vi "OSA_example_XYarray.vi"() -> ()   [LabVIEW 2010]
doc: "Example of how to create the X-data if not present after acquisition."
uses:
  _OSA_class/OSA.lvclass
  _OSA_class/typeDef/acq_dataType.ctl
  _misc/Thorlabs_FTS_misc.llb/graph_spectrum.ctl
  OSA20X_misc.lvlib
panel:
  out "timeOut":bool
  in  "X-UNIT":T1(ring)=enum."NM_VAC"
  out "Intensity Graph spectrum":T2
  in  "virtual OSA":bool=TRUE
  out "X,Y (row 0,1)":sgl[][](array[numeric])
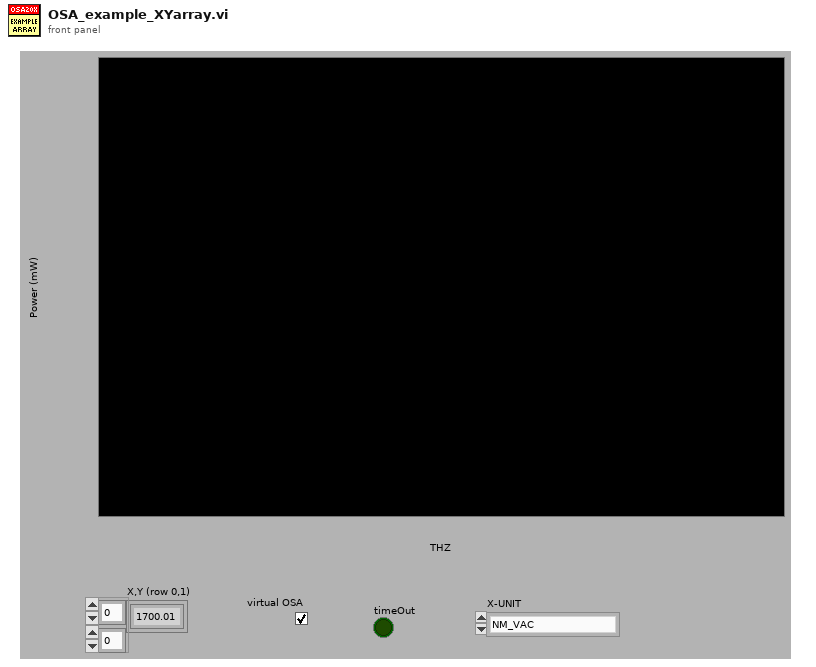
[diagram p1: front panel]
types:
  T1 = enum16{"WAVENR/CM", "EV", "THZ", "NM_AIR", "NM_VAC"}
  T2 = typedef "OSA20X_misc.lvlib/graph_spectrum.ctl" = i32[][]
  T3 = enum16{"OSA201", "OSA202", "OSA203", "OSA204", "OSA205", "OSA206", "OSA207", "OSA208"}
  T4 = cluster{"waveCenter (nm)":dbl, "FWHM (nm)":dbl, "peakAmplitude":dbl}
  T5 = typedef "OSA.lvclass/acq_dataType.ctl" = enum16{"none", "interferogram", "spectrum"}
  T6 = typedef "OSA.lvclass/xVal_option.ctl" = enum16{"MIN_MAX", "ARRAY"}
  T7 = cluster{"length":u32, "X min":sgl, "X max":sgl, "X_VAL_OPTIONS":T6}
  T8 = enum16{"pressure", "temperature", "humidity", "all"}
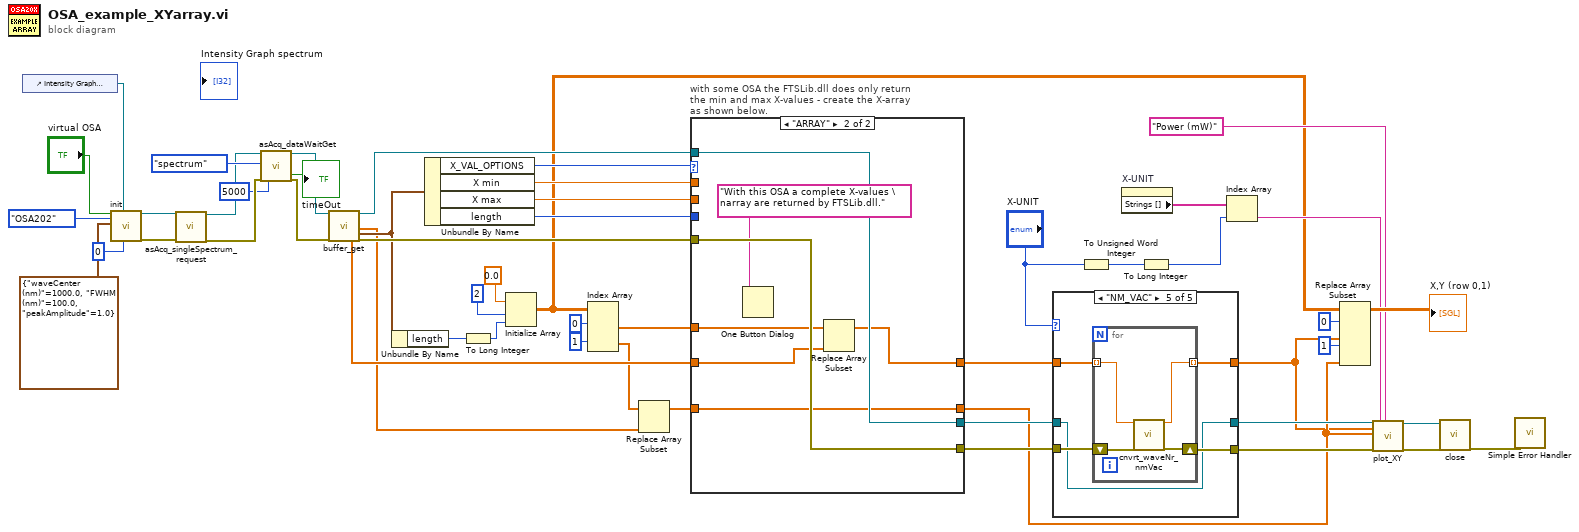
[diagram p0: block diagram]
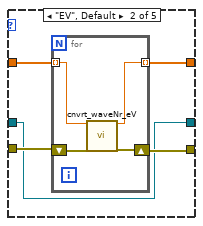
[diagram p3: hidden frame]
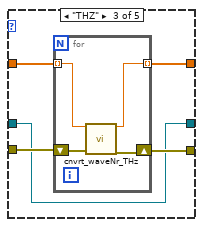
[diagram p4: hidden frame]
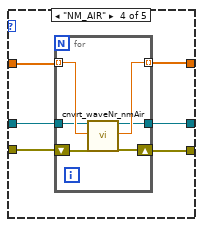
[diagram p5: hidden frame]
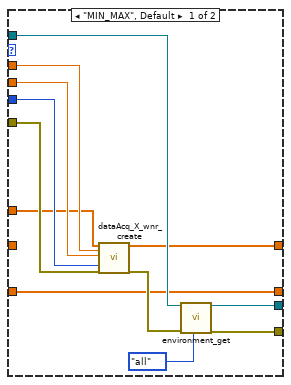
[diagram p6: hidden frame]
diagram:
  n1 = control-ref of="Intensity Graph spectrum"() -> (w21:refnum<vi>)
  n2 = call "init.vi"("virtual OSA"="virtual OSA", "virtual OSA model"=T3."OSA202", "virtual OSA source"=T4 {"waveCenter (nm)"=1000.0, "FWHM (nm)"=100.0, "peakAmplitude"=1.0}, "Graph Spectrum"=w21, "spectrIdx"=u16 0) -> ("duplicate reference"=w34:refnum<class "OSA.lvclass">, "error out"=w35:errorcluster)  [unwired: 10 in, 3 out]
  n3 = call "asAcq_singleSpectrum_request.vi"("reference"=w34, "error in (no error)"=w35) -> ("duplicate reference"=w33:refnum<class "OSA.lvclass">, "error out"=w32:errorcluster)  [unwired: 16 in]
  n4 = call "asAcq_dataWaitGet.vi"("reference"=w33, "dataType"=acq_dataType."spectrum", "error in (no error)"=w32, "timeout (20000 ms)"=5000) -> ("timeOut"=→"timeOut":bool, "duplicate reference"=w52:refnum<class "OSA.lvclass">, "error out"=w51:errorcluster)  [unwired: 12 in, 1 out]
  n5 = call-dynamic "buffer_get.vi"("reference in"=w52, "error in (no error)"=w51) -> ("spectrum X, (wavenr/cm)"=w27:sgl[], "reference out"=w38:refnum<class "OSA.lvclass">, "spectrum Y (mW)"=w6:sgl[], "spectrum properties"=w44:T7, "error out"=w45:errorcluster)  [unwired: 11 in, 2 out]
  n6 = Unbundle By Name(w44) -> ("length"=w47:u32)
  n7 = Unbundle By Name(w44) -> ("X_VAL_OPTIONS"=w28:T6, "X min"=w41:sgl, "X max"=w40:sgl, "length"=w39:u32)
  n8 = To Long Integer(number=w47) -> (32bit integer=w48:i32)
  n9 = Initialize Array(sgl 0.0 ("element"), 2 ("dimension size"), w48) -> (w1:sgl[][])
  n10 = Index Array(array=w1, index (row) #1=0 ("index (row)"), index (row) #2=1 ("index (row)")) -> (element #1=w4:sgl[], element #2=w7:sgl[])  [unwired: 2 in]
  n11 = Replace Array Subset(array=w7, new element=w6) -> (w5:sgl[])  [unwired: 1 in]
  n12 = case "with some OSA the FTSLib.dll does only return the min and max X-values - create the X-array as shown below." shown="\"ARRAY\"" w28 {
    tunnel: w45 -> [w64 w71]
    tunnel: w41 -> [w63 _]
    tunnel: w40 -> [w62 _]
    tunnel: w39 -> [w61 _]
    tunnel: w38 -> [w59 w70]
    tunnel: [w55 w70] -> w25
    tunnel: [w56 w71] -> w26
    tunnel: [w57 w65] -> w24
    tunnel: w27 -> [_ w66]
    tunnel: w5 -> [w54 w68]
    tunnel: w4 -> [w53 w67]
    tunnel: [w54 w68] -> w3
    frame "MIN_MAX", Default {
      n13 = call "dataAcq_X_wnr_create.vi"("x scale in, (WNr, THz, )"=w53, "x_min"=w63, "x_max"=w62, "points"=w61, "error in (no error)"=w64) -> ("x scale out"=w57:sgl[], "error out"=w60:errorcluster)  [unwired: 13 in]
      n14 = call "environment_get.vi"("reference"=w59, "error in (no error)"=w60, "parameter"=T8."all") -> ("duplicate reference"=w55:refnum<class "OSA.lvclass">, "error out"=w56:errorcluster)  [unwired: 9 in, 6 out]
    }
    frame "ARRAY" {
      n15 = One Button Dialog(message="With this OSA a complete X-values \narray are returned by FTSLib.dll.") -> ()  [unwired: 1 in, 1 out]
      n16 = Replace Array Subset(array=w67, new element=w66) -> (w65:sgl[])  [unwired: 1 in]
    }
  }
  n17 = case shown="\"NM_VAC\"" "X-UNIT" {
    tunnel: w25 -> [w73 w75 w84 w95 w105]
    tunnel: w26 -> [w72 w79 w88 w98 w107]
    tunnel: w24 -> [w74 w78 w87 w97 w109]
    tunnel: [w74 w77 w86 w96 w108] -> w2
    tunnel: [w73 w75 w84 w94 w105] -> w17
    tunnel: [w72 w76 w85 w93 w106] -> w20
    frame "WAVENR/CM" {
    }
    frame "EV", Default {
      n18 = for {
        shift-right: [w82] -> w76
        shift-left: w79 -> [w83]
        tunnel: w78 -> [w81] mode=indexing
        tunnel: [w80] -> w77 mode=indexing
        n19 = call "cnvrt_waveNr_eV.vi"("waveNr"=w81, "error in (no error)"=w83) -> ("energy (eV)"=w80:dbl, "error out"=w82:errorcluster)  [unwired: 16 in]
      }
    }
    frame "THZ" {
      n20 = for {
        shift-right: [w91] -> w85
        shift-left: w88 -> [w92]
        tunnel: w87 -> [w90] mode=indexing
        tunnel: [w89] -> w86 mode=indexing
        n21 = call "cnvrt_waveNr_THz.vi"("waveNr"=w90, "error in (no error)"=w92) -> ("frequency (THz)"=w89:dbl, "error out"=w91:errorcluster)  [unwired: 16 in]
      }
    }
    frame "NM_AIR" {
      n22 = for {
        shift-right: [w103] -> w93
        shift-left: w98 -> [w104]
        tunnel: w97 -> [w102] mode=indexing
        tunnel: [w101] -> w96 mode=indexing
        tunnel: w95 -> [w100]
        tunnel: [w99] -> w94
        n23 = call "cnvrt_waveNr_nmAir.vi"("reference in"=w100, "waveNr"=w102, "error in (no error)"=w104) -> ("reference out"=w99:refnum<class "OSA.lvclass">, "wavelength (nmAir)"=w101:dbl, "error out"=w103:errorcluster)  [unwired: 14 in]
      }
    }
    frame "NM_VAC" {
      n24 = for {
        tunnel: w109 -> [w113] mode=indexing
        tunnel: [w112] -> w108 mode=indexing
        shift-right: [w110] -> w106
        shift-left: w107 -> [w111]
        n25 = call "cnvrt_waveNr_nmVac.vi"("waveNr"=w113, "error in (no error)"=w111) -> ("wavelength (nmVac)"=w112:dbl, "error out"=w110:errorcluster)  [unwired: 16 in]
      }
    }
  }
  n26 = To Unsigned Word Integer(number="X-UNIT") -> (unsigned 16bit integer=w14:u16)
  n27 = property on="X-UNIT" class="Enum (strict)"() -> ("Strings []"=w16:string[])  [unwired: 2 in, 2 out]
  n28 = To Long Integer(number=w14) -> (32bit integer=w13:i32)
  n29 = Index Array(array=w16, index=w13) -> (element=w12:string)
  n30 = Replace Array Subset(array=w1, new element #1=w2, index (row) #1=0 ("index (row)"), new element #2=w3, index (row) #2=1 ("index (row)")) -> (→"X,Y (row 0,1)":sgl[][])  [unwired: 2 in]
  n31 = call "plot_XY.vi"("reference"=w17, "X-data"=w2, "Y-data"=w3, "error in (no error)"=w20, "Label X-scale"=w12, "Label Y-scale"="Power (mW)") -> ("duplicate reference"=w18:refnum<class "OSA.lvclass">, "error out"=w19:errorcluster)  [unwired: 12 in]
  n32 = call "close.vi"("reference"=w18, "error in (no error)"=w19) -> ("error out"=w36:errorcluster)  [unwired: 17 in]
  n33 = call <vilib>:"Simple Error Handler.vi"("error in (no error)"=w36) -> ()  [unwired: 4 in, 5 out]
